vi "part_2.vi"() -> ()   [LabVIEW 2020]
panel:
  in  "Enable Channel 1 to 3":bool
  in  "Channel List ({Channel1}) 2":i32[](array[ring])=[0] items=["Channel 1", "Channel 2"]
  out "resulting string":string
  in  "Device Action (2: Both)":i32(ring)=2 items=["Acquire", "Transient", "Both"]
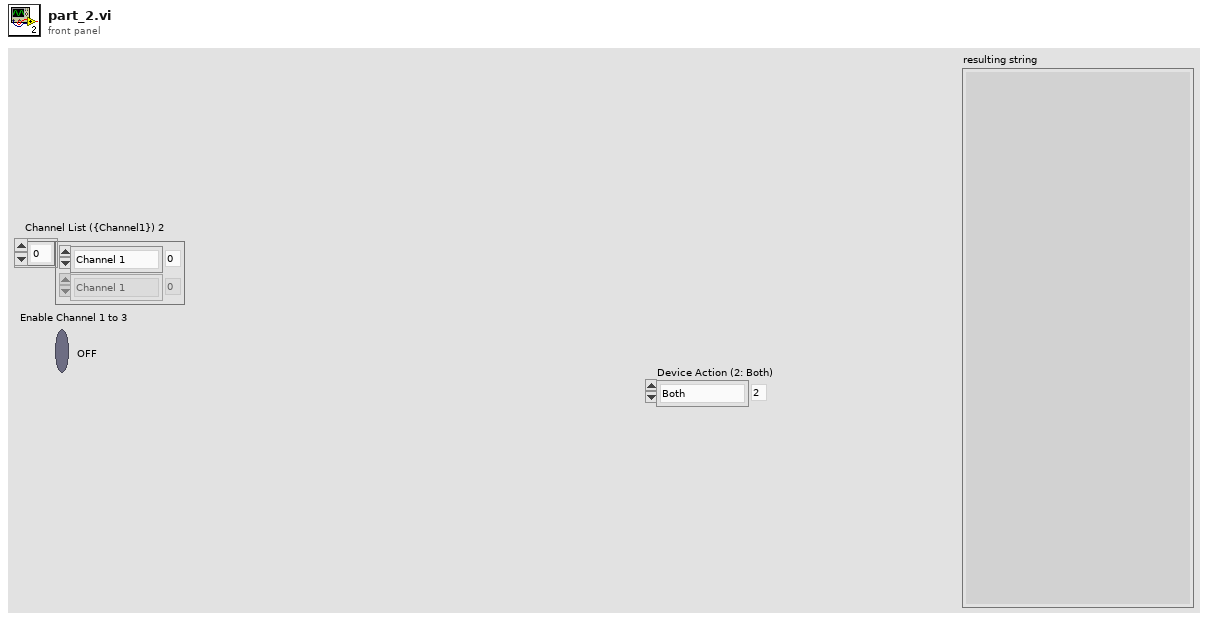
[diagram p1: front panel]
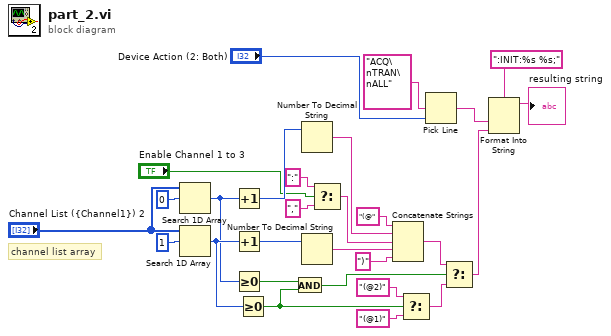
[diagram p0: block diagram]
diagram:
  # "channel list array"
  n1 = Search 1D Array(1D array="Channel List ({Channel1}) 2", element=0) -> (index of element=w10:i32)  [unwired: 1 in]
  n2 = Search 1D Array(1D array="Channel List ({Channel1}) 2", element=1) -> (index of element=w12:i32)  [unwired: 1 in]
  n3 = Increment(x=w10) -> (x+1=w9:i32)
  n4 = Increment(x=w12) -> (x+1=w11:i32)
  n5 = Greater Or Equal To 0?(x=w10) -> (x >= 0?=w20:bool)
  n6 = Greater Or Equal To 0?(x=w12) -> (x >= 0?=w18:bool)
  n7 = And(x=w20, y=w18) -> (x .and. y?=w19:bool)
  n8 = Number To Decimal String(number=w9) -> (decimal integer string=w6:string)  [unwired: 1 in]
  n9 = Number To Decimal String(number=w11) -> (decimal integer string=w5:string)  [unwired: 1 in]
  n10 = Select(t=":", s="Enable Channel 1 to 3", f=",") -> (s? t:f=w8:string)
  n11 = Concatenate Strings("(@", w6, w8, w5, ")") -> (w3:string)
  n12 = Select(t="(@2)", s=w18, f="(@1)") -> (s? t:f=w15:string)
  n13 = Pick Line(multi-line string="ACQ\nTRAN\nALL", line index="Device Action (2: Both)") -> (output string=w25:string)  [unwired: 1 in]
  n14 = Select(t=w3, s=w19, f=w15) -> (s? t:f=w1:string)
  n15 = Format Into String(format string=":INIT:%s %s;", w25, w1) -> (resulting string=→"resulting string":string)  [unwired: 2 in, 1 out]
